vi "shutter.vi"(8 "error in (no error)":errorcluster, 9 "servo":i32(ring) items=["ServoUnspecified", "ServoCh1", "ServoCh2", "ServoBoth"], 10 "Status":bool, 11 "channel":refnum<k24>) -> (0 "error out":errorcluster)   [LabVIEW 2021]
uses:
  F:/2PhotonVision/psychometric_function_v2/lib/Grpc.Core.dll
  lib/Grpc.Core.dll
  F:/2PhotonVision/psychometric_function_v2/lib/FossilProtosSharp.dll
  lib/FossilProtosSharp.dll
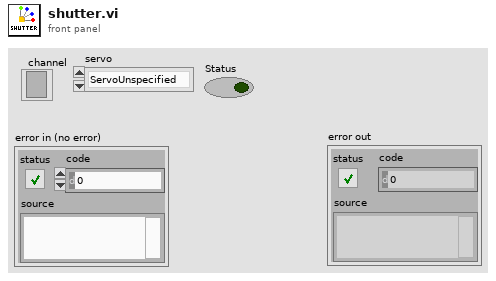
[diagram p1: front panel]
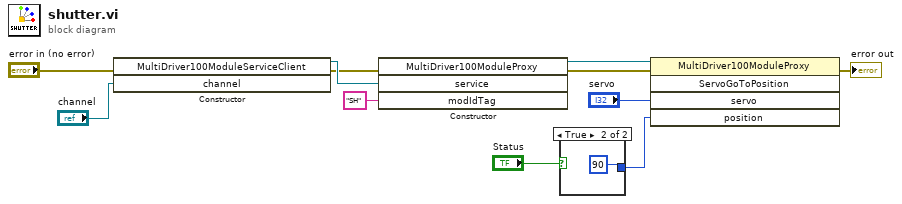
[diagram p0: block diagram]
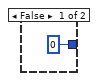
[diagram p2: hidden frame]
diagram:
  n1 = constructor class="MultiDriver100ModuleServiceClie"(error in="error in (no error)", "channel"="channel") -> (reference out=w9:refnum<k24>, error out=w8:errorcluster)  [unwired: 2 in, 2 out]
  n2 = constructor class="MultiDriver100ModuleProxy"(error in=w8, "service"=w9, "modIdTag"="SH") -> (reference out=w5:refnum<k24>, error out=w4:errorcluster)  [unwired: 2 in, 3 out]
  n3 = case shown="True" "Status" {
    tunnel: [0 90] -> w2
    frame False {
    }
    frame True {
    }
  }
  n4 = invoke class="MultiDriver100ModuleProxy" method="ServoGoToPosition"(reference=w5, error in=w4, "servo"="servo", "position"=w2) -> (error out=→"error out":errorcluster)  [unwired: 1 in, 4 out]
